vi "PrintVIDocumentation.vi"(10 "HTML Target Dir":path, 11 "Folder Path":path) -> (0 "error out":errorcluster, 2 "Progress %":dbl, 3 "Number of Files":i32, 9 "All Files in Dir":path[](array[path]))   [LabVIEW 2019]
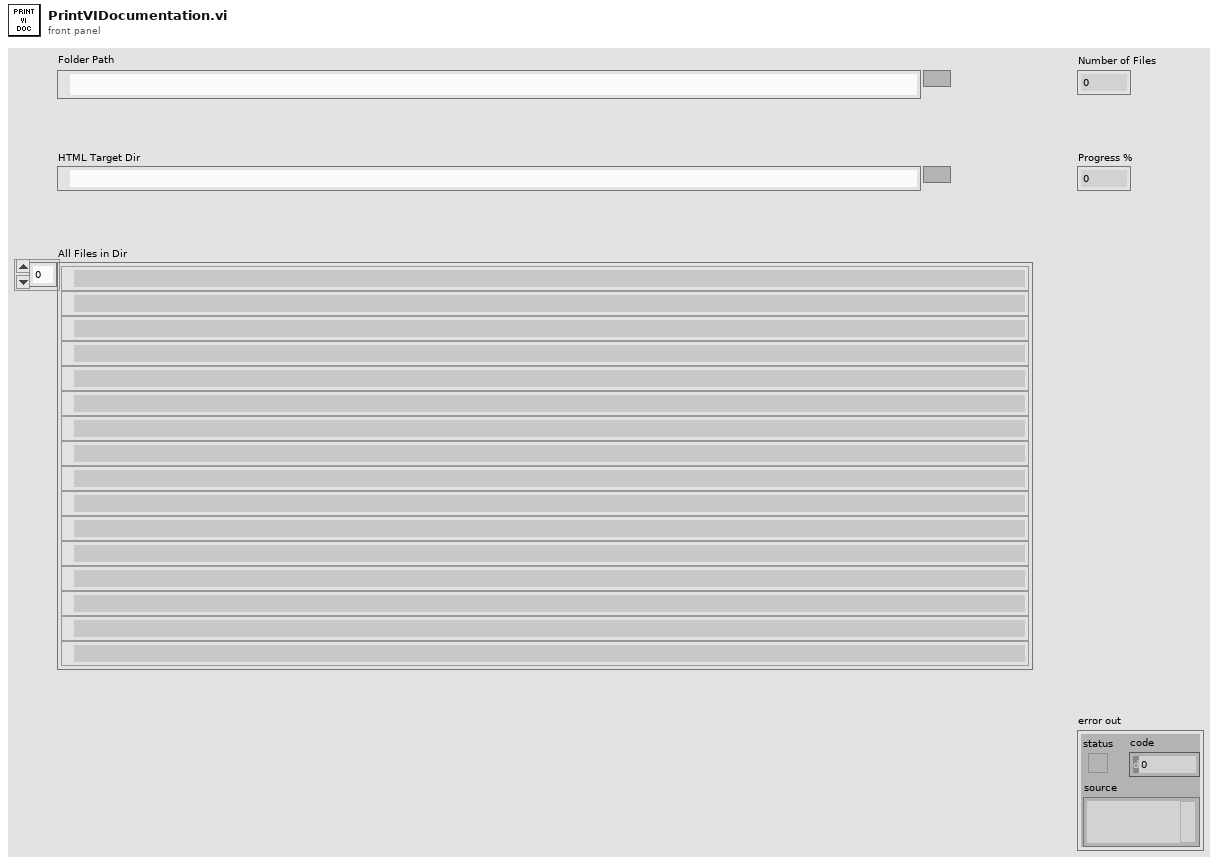
[diagram p1: front panel]
types:
  T1 = enum32{"Custom", "Standard", "Using Panel", "Using SubVI", "Complete"}
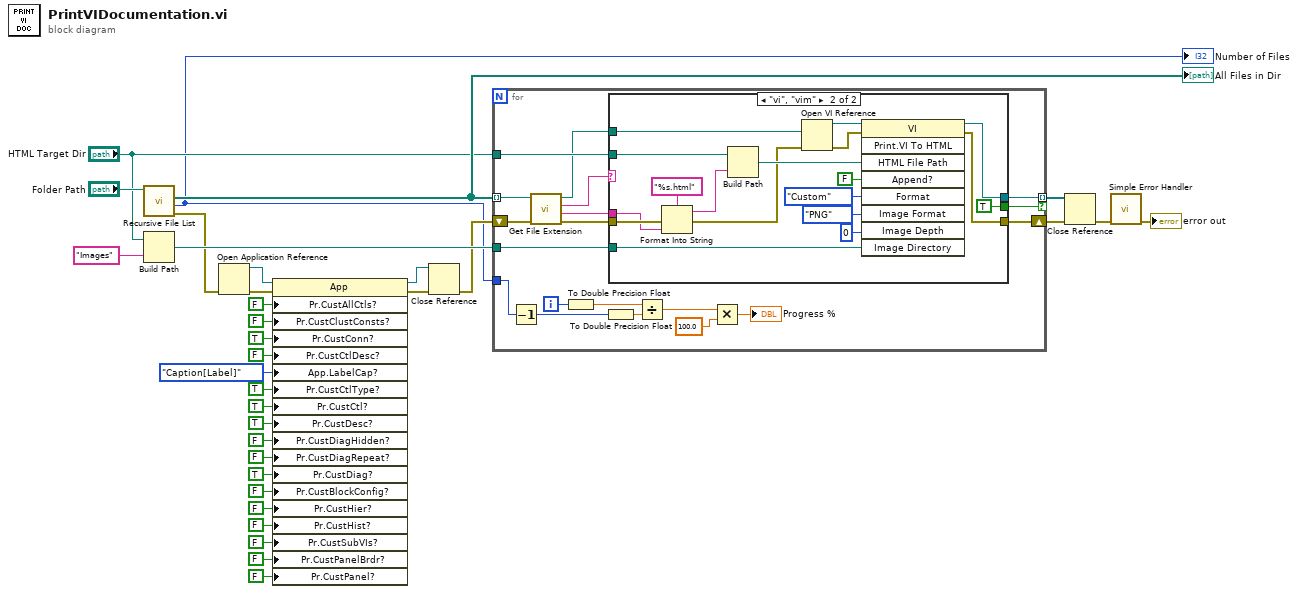
[diagram p0: block diagram]
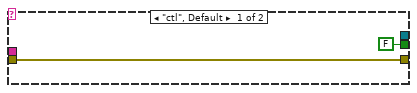
[diagram p2: hidden frame]
diagram:
  n1 = call <vilib>:"Recursive File List.vi"("Folder Path"="Folder Path") -> ("error out"=w23:errorcluster, "Number of Files"=w4:i32, "All Files in Dir"=w32:path[])  [unwired: 6 in, 2 out]
  "All Files in Dir" <- w32
  "Number of Files" <- w4
  n2 = Build Path(base path="HTML Target Dir", name or relative path="Images") -> (appended path=w29:path)
  n3 = Open Application Reference(8:w23) -> (0:w27:errorcluster, 3:w28:refnum<vi>)  [unwired: 3 in]
  n4 = property class="App"(reference=w28, error in=w27, "Pr.CustAllCtls?"=FALSE ("Printing:Custom All Controls?"), "Pr.CustClustConsts?"=FALSE ("Printing:Custom Cluster Constants?"), "Pr.CustConn?"=TRUE ("Printing:Custom Connector?"), "Pr.CustCtlDesc?"=FALSE ("Printing:Custom Control Descriptions?"), "App.LabelCap?"=enum16{"Label", "Caption", "Caption[Label]"}."Caption[Label]" ("Printing:Custom Control Label/Caption?"), "Pr.CustCtlType?"=TRUE ("Printing:Custom Control Types?"), "Pr.CustCtl?"=TRUE ("Printing:Custom Controls?"), "Pr.CustDesc?"=TRUE ("Printing:Custom Description?"), "Pr.CustDiagHidden?"=FALSE ("Printing:Custom Diagram Hidden?"), "Pr.CustDiagRepeat?"=FALSE ("Printing:Custom Diagram Repeat?"), "Pr.CustDiag?"=TRUE ("Printing:Custom Diagram?"), "Pr.CustBlockConfig?"=FALSE ("Printing:Custom Express VI Configuration?"), "Pr.CustHier?"=FALSE ("Printing:Custom Hierarchy?"), "Pr.CustHist?"=FALSE ("Printing:Custom History?"), "Pr.CustSubVIs?"=FALSE ("Printing:Custom List of SubVIs?"), "Pr.CustPanelBrdr?"=FALSE ("Printing:Custom Panel Border?"), "Pr.CustPanel?"=FALSE ("Printing:Custom Panel?")) -> (reference out=w24:refnum<vi>, error out=w26:errorcluster)
  n5 = Close Reference(reference=w24, error in (no error)=w26) -> (error out=w25:errorcluster)
  n6 = for {
    tunnel: w32 -> [w49] mode=indexing
    shift-right: [w42] -> w2
    shift-left: w25 -> [w50]
    tunnel: "HTML Target Dir" -> [w51]
    tunnel: w29 -> [w52]
    tunnel: w4 -> [w45]
    tunnel: [w43] -> w3 mode=indexing if=w36
    i -> [w40]
    n7 = Decrement(x=w45) -> (x-1=w41:i32)
    n8 = call <vilib>:"Get File Extension.vi"("error in (no error)"=w50, "file"=w49) -> ("error out"=w48:errorcluster, "filename without extension"=w46:string, "lowercase file extension"=w44:string, "dup file"=w47:path)  [unwired: 5 in, 1 out]
    n9 = To Double Precision Float(number=w40) -> (double precision float=w38:dbl)
    n10 = To Double Precision Float(number=w41) -> (double precision float=w39:dbl)
    n11 = case shown="\"vi\", \"vim\"" w44 {
      tunnel: w52 -> [_ w67]
      tunnel: w51 -> [_ w65]
      tunnel: w48 -> [w54 w62]
      tunnel: w47 -> [_ w60]
      tunnel: w46 -> [_ w59]
      tunnel: [w54 w57] -> w42
      tunnel: [_ w56] -> w43
      tunnel: [FALSE TRUE] -> w36
      frame "ctl", Default {
      }
      frame "vi", "vim" {
        n12 = Format Into String(format string="%s.html", error in=w62, w59) -> (resulting string=w63:string, error out=w61:errorcluster)  [unwired: 1 in]
        n13 = Build Path(base path=w65, name or relative path=w63) -> (appended path=w64:path)
        n14 = Open VI Reference(vi path=w60, error in (no error)=w61) -> (vi reference=w72:refnum<vi>, error out=w71:errorcluster)  [unwired: 4 in]
        n15 = invoke class="VI" method="Print.VI To HTML"(reference=w72, error in=w71, "HTML File Path"=w64, "Append?"=FALSE, "Format"=T1."Custom", "Image Format"=enum32{"PNG", "JPEG", "GIF"}."PNG", "Image Depth"=0, "Image Directory"=w67) -> (reference out=w56:refnum<vi>, error out=w57:errorcluster)  [unwired: 1 in, 7 out]
      }
    }
    n16 = Divide(x=w38, y=w39) -> (x/y=w37:dbl)
    n17 = Multiply(x=w37, y=100.0 ("x")) -> (x*y=→"Progress %":dbl)
  }
  n18 = Close Reference(reference=w3, error in (no error)=w2) -> (error out=w1:errorcluster)
  n19 = call <vilib>:"Simple Error Handler.vi"("error in (no error)"=w1) -> ("error out"=→"error out":errorcluster)  [unwired: 4 in, 4 out]
